vi "Compare Index Signature.vi"(8 "error in (no error)":errorcluster, 11 "Indexing Test Finder in":refnum<class "Indexing Test Finder.lvclass">) -> (0 "error out":errorcluster, 3 "Indexing Test Finder out":refnum<class "Indexing Test Finder.lvclass">)   [LabVIEW 2020, in "Indexing Test Finder.lvclass"]
doc: "Compares signture of index to the actual class library to detect changes.\nThe signare in the index is updated to match the library if there is a missmatch."
uses:
  Indexing Test Finder.lvclass
  <vilib>/Utility/miscctls.llb/LVMapReplaceAction.ctl
  Test Finder/Test Finder.lvclass
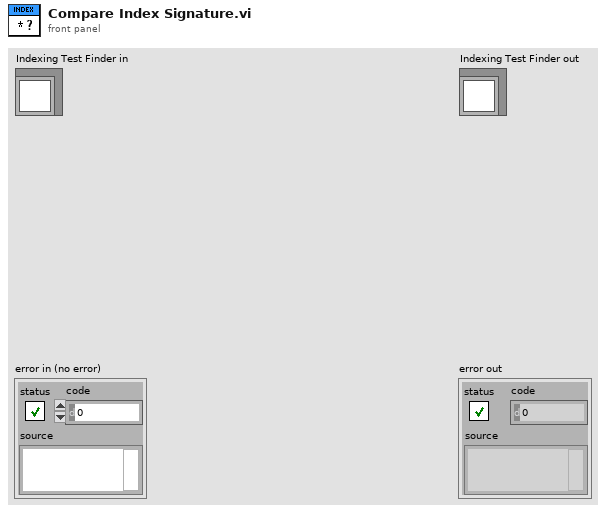
[diagram p1: front panel]
types:
  T1 = typedef "LVMapReplaceAction.ctl" = enum32{"Modify Entry only if found", "Add or Modify Entry", "Delete Entry"}
  T2 = typedef "Indexing Test Finder.lvclass/Index Item.ctl" = cluster{"Dynamic Methods":map{string, path}, "Static Methods":map{string, path}, "Signature":string}
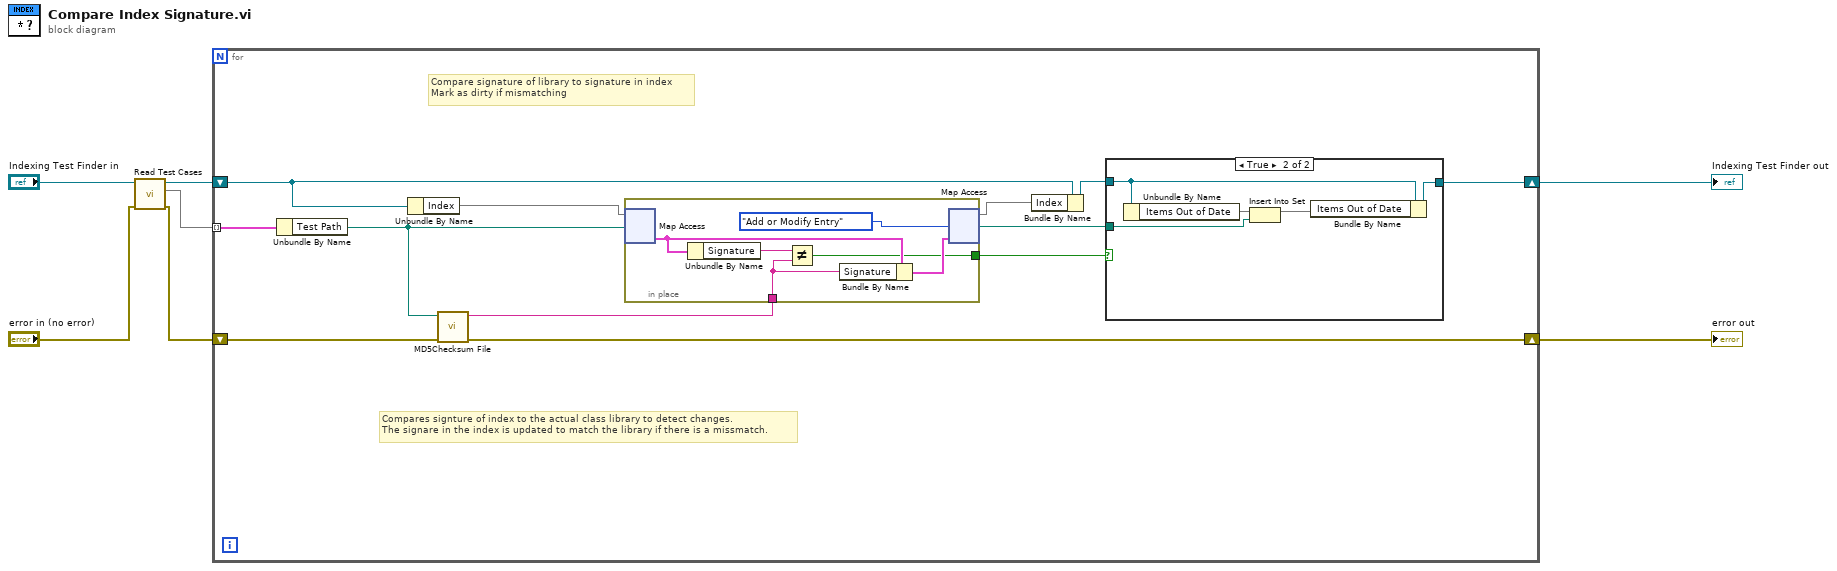
[diagram p0: block diagram]
diagram:
  n1 = call "Read Test Cases.vi"("error in (no error)"="error in (no error)", "Test Finder In"="Indexing Test Finder in") -> ("error out"=w2:errorcluster, "Test Cases"=w3:map{string, path}, "Test Finder Out"=w4:refnum<class "Indexing Test Finder.lvclass">)  [unwired: 7 in]
  n2 = for {
    tunnel: w3 -> [w13] mode=indexing
    shift-right: [w10] -> w5
    shift-left: w2 -> [w11]
    shift-right: [w19] -> w6
    shift-left: w4 -> [w9]
    # "Compares signture of index to the actual class library to detect changes.\nThe signare in the index is updated to match the library if there is a missmatch."
    # "Compare signature of library to signature in index\nMark as dirty if mismatching"
    n3 = Unbundle By Name(w13) -> ("Test Path"=w8:path)
    n4 = Unbundle By Name(w9) -> ("Index"=w18:map{path, T2})
    n5 = call <vilib>:"MD5Checksum File.vi"("error in (no error)"=w11, "Path"=w8) -> ("error out"=w10:errorcluster, "MD5 message-digest"=w12:string)  [unwired: 8 in]
    n6 = in-place {
      in-place-border: w12 -> [w29]
      in-place-border: [w26] -> w16
      n7 = in-place-map #1(w18, w8) -> (w31:T2)  [unwired: 1 in, 1 out]
      n8 = Unbundle By Name(w31) -> ("Signature"=w30:string)
      n9 = Not Equal?(x=w30, y=w29) -> (x != y?=w26:bool)
      n10 = Bundle By Name(cluster=w31, "Signature"=w29) -> (w28:T2)
      n11 = in-place-map #1(w28, LVMapReplaceAction."Add or Modify Entry" ("action")) -> (w14:map{path, T2}, w17:path)  [unwired: 1 out]
    }
    n12 = Bundle By Name(cluster=w9, "Index"=w14) -> (w15:refnum<class "Indexing Test Finder.lvclass">)
    n13 = case shown="True" w16 {
      tunnel: w15 -> [w20 w25]
      tunnel: [w20 w24] -> w19
      tunnel: w17 -> [_ w21]
      frame False {
      }
      frame True {
        n14 = Unbundle By Name(w25) -> ("Items Out of Date"=w23:set{path})
        n15 = Insert Into Set(10:w21, 11:w23) -> (3:w22:set{path})  [unwired: 1 out]
        n16 = Bundle By Name(cluster=w25, "Items Out of Date"=w22) -> (w24:refnum<class "Indexing Test Finder.lvclass">)
      }
    }
  }
  "error out" <- w5
  "Indexing Test Finder out" <- w6
